vi "createDigitalOutTask.vi"(8 "error in":errorcluster, 11 "daq_do":tag="Dev1/ai0:1") -> (0 "error out":errorcluster, 3 "task out":refnum<k21>)   [LabVIEW 2019]
uses:
  <vilib>/DAQmx/create/channels.llb/DAQmx Create Channel (DO-Digital Output).vi
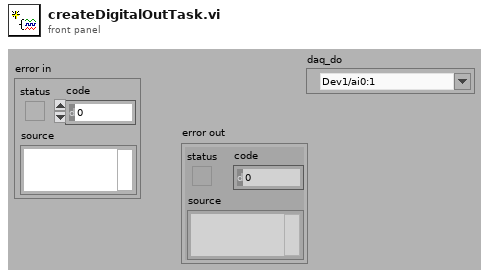
[diagram p1: front panel]
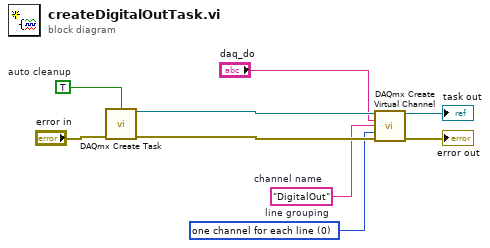
[diagram p0: block diagram]
diagram:
  w5 = 0 items=["one channel for each line", "one channel for all lines"]  # line grouping
  w4 = "DigitalOut"  # channel name
  w7 = TRUE  # auto cleanup
  n1 = call <vilib>:"DAQmx Create Task.vi"("auto cleanup"=w7, "error in"="error in") -> ("task out"=w6:refnum<k21>, "error out"=w8:errorcluster)  [unwired: 12 in]
  n2 = call-poly <vilib>:"DAQmx Create Virtual Channel.vi"("task in"=w6, "lines"="daq_do", "name to assign"=w4, "line grouping"=w5, "error in"=w8) -> ("task out"=→"task out":refnum<k21>, "error out"=→"error out":errorcluster)  [unwired: 9 in]
